vi "模板建立.vi"(1 "输入信号特征参数":dbl[][](array[numeric]), 2 "Path":path) -> (0 "输出信号特征参数":dbl[][](array[numeric]))   [LabVIEW 2018]
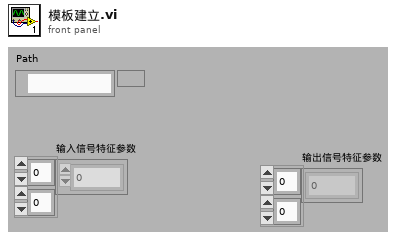
[diagram p1: front panel]
types:
  T1 = enum16{"open", "replace", "create", "open or create", "replace or create", "replace or create with confirmation"}
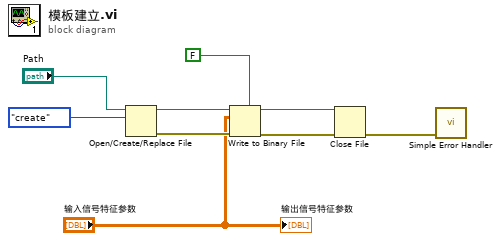
[diagram p0: block diagram]
diagram:
  n1 = Open/Create/Replace File(file path (use dialog)="Path", operation (0:open)=T1."create") -> (refnum out=w4:refnum<file>, error out=w7:errorcluster)  [unwired: 4 in, 1 out]
  n2 = Write to Binary File(file (use dialog)=w4, data="输入信号特征参数", error in=w7, 5:FALSE ("prepend array or string size? (T)")) -> (refnum out=w3:refnum<file>, error out=w8:errorcluster)  [unwired: 2 in, 1 out]
  n3 = Close File(refnum=w3, error in=w8) -> (error out=w9:errorcluster)  [unwired: 1 out]
  n4 = call <vilib>:"Simple Error Handler.vi"("error in (no error)"=w9) -> ()  [unwired: 4 in, 5 out]
  "输出信号特征参数" <- "输入信号特征参数"
